vi "Start ssh-agent.vi"(8 "error in (no error)":errorcluster, 11 "Agent Fixture in":refnum<class "Agent Fixture.lvclass">) -> (0 "error out":errorcluster, 3 "Agent Fixture out":refnum<class "Agent Fixture.lvclass">)   [LabVIEW 2013, in "libssh2_integration_tests.lvlib" / "Agent Fixture.lvclass"]
uses:
  Agent Fixture.lvclass
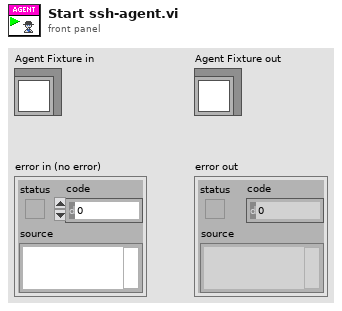
[diagram p1: front panel]
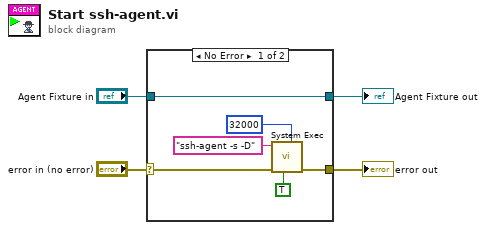
[diagram p0: block diagram]
diagram:
  n1 = case shown="No Error" "error in (no error)" {
    selector: "error in (no error)" -> [w10 w12]
    tunnel: [w9 w12] -> w3
    tunnel: [w8 w11] -> w1
    tunnel: "Agent Fixture in" -> [w8 w11]
    frame No Error {
      n2 = call <vilib>:"System Exec.vi"("expected output size  (4096)"=u32 32000, "run minimized? (F)"=TRUE, "error in (no error)"=w10, "command line"="ssh-agent -s -D") -> ("error out"=w9:errorcluster)  [unwired: 4 in, 3 out]
    }
    frame Error {
    }
  }
  "error out" <- w3
  "Agent Fixture out" <- w1
